vi "Flywheel Speed.vi"(11 "Distance Type":enum16{"SONAR", "VISION", "BOTH"}(ring)) -> (1 "Calculation_Ready":bool, 2 "In_Range":bool, 3 "Suggested Speed":dbl)   [LabVIEW 2015]
uses:
  <vilib>/Analysis/baseanly.llb/Mean (DBL).vi
  Robot Global Data.vi
  <vilib>/Analysis/NI_AALPro.lvlib
  <vilib>/Analysis/NI_AALBase.lvlib
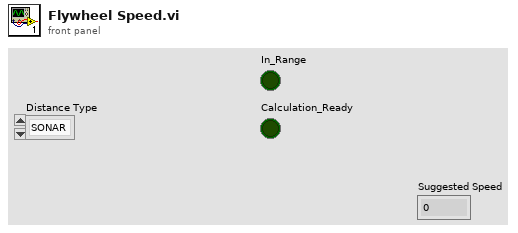
[diagram p1: front panel]
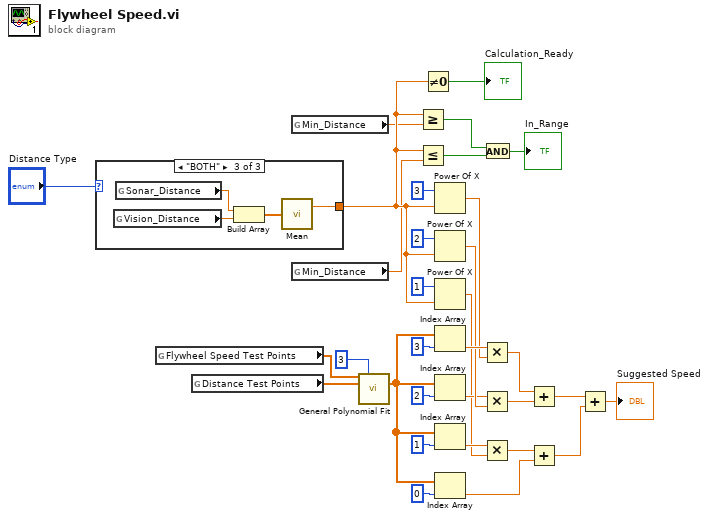
[diagram p0: block diagram]
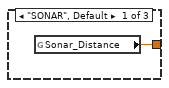
[diagram p2: hidden frame]
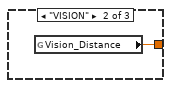
[diagram p3: hidden frame]
diagram:
  n1 = case shown="\"BOTH\"" "Distance Type" {
    tunnel: [w33 w34 w35] -> w5
    frame "SONAR", Default {
      n2 = global read "Robot Global Data.vi" "Sonar_Distance"() -> (w33:dbl)
    }
    frame "VISION" {
      n3 = global read "Robot Global Data.vi" "Vision_Distance"() -> (w34:dbl)
    }
    frame "BOTH" {
      n4 = global read "Robot Global Data.vi" "Vision_Distance"() -> (w38:dbl)
      n5 = global read "Robot Global Data.vi" "Sonar_Distance"() -> (w37:dbl)
      n6 = Build Array(w37, w38) -> (w36:dbl[])
      n7 = call-poly <vilib>:"Mean.vi"("X"=w36) -> ("mean"=w35:dbl)  [unwired: 1 out]
    }
  }
  n8 = global read "Robot Global Data.vi" "Flywheel Speed Test Points"() -> (w1:dbl[])
  n9 = global read "Robot Global Data.vi" "Distance Test Points"() -> (w2:dbl[])
  n10 = global read "Robot Global Data.vi" "Min_Distance"() -> (w3:dbl)
  n11 = global read "Robot Global Data.vi" "Min_Distance"() -> (w4:dbl)
  n12 = call <vilib>:"General Polynomial Fit.vi"("Y"=w1, "polynomial order"=3, "X"=w2) -> ("Polynomial Coefficients"=w23:dbl[])  [unwired: 9 in, 3 out]
  n13 = Greater Or Equal?(x=w5, y=w3) -> (x >= y?=w9:bool)
  n14 = Less Or Equal?(x=w5, y=w4) -> (x <= y?=w8:bool)
  n15 = Not Equal To 0?(x=w5) -> (x != 0?=→"Calculation_Ready":bool)
  n16 = Power Of X(1:w5, 2:3) -> (0:w26:dbl)
  n17 = Power Of X(1:w5, 2:2) -> (0:w25:dbl)
  n18 = Power Of X(1:w5, 2:1) -> (0:w21:dbl)
  n19 = Index Array(array=w23, index=3) -> (element=w27:dbl)
  n20 = Index Array(array=w23, index=2) -> (element=w24:dbl)
  n21 = Index Array(array=w23, index=1) -> (element=w22:dbl)
  n22 = Index Array(array=w23, index=0) -> (element=w18:dbl)
  n23 = Multiply(x=w27, y=w26) -> (x*y=w20:dbl)
  n24 = Multiply(x=w24, y=w25) -> (x*y=w19:dbl)
  n25 = Multiply(x=w22, y=w21) -> (x*y=w17:dbl)
  n26 = And(x=w9, y=w8) -> (x .and. y?=→"In_Range":bool)
  n27 = Add(x=w20, y=w19) -> (x+y=w16:dbl)
  n28 = Add(x=w17, y=w18) -> (x+y=w15:dbl)
  n29 = Add(x=w16, y=w15) -> (x+y=→"Suggested Speed":dbl)
